vi "Execution Closed Event Callback.vi"(4 "TS UI Data":T1, 5 "Event Data":cluster{"exec":refnum<k7>}, 6 "Control Ref":refnum<k7>, 7 "Event Common Data":T2) -> ()   [LabVIEW 2015]
uses:
  Type defs/TS UI Data.ctl
  Type defs/Nest cluster.ctl
panel:
  # "SCANNED DATA"
  # "ITAC DATA"
  # "DoIP DATA"
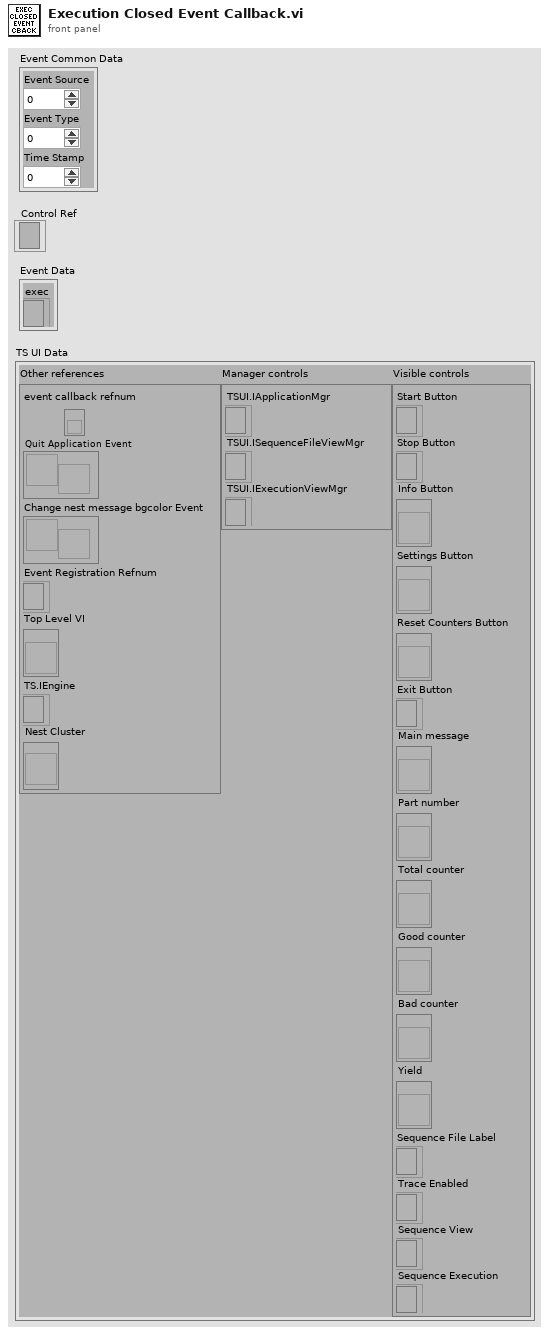
[diagram p1: front panel]
types:
  T1 = typedef "TS UI Data.ctl" = cluster{"Other references":cluster{"event callback refnum":refnum<k27>, "Quit Application Event":refnum<user-event>, "Change nest message bgcolor Event":refnum<user-event>, "event registration refnum":refnum<event-registration>, "Top Level VI":refnum<vi>, "TS.IEngine":refnum<k7>, "Nest Cluster":refnum<vi>}, "Manager controls":cluster{"TSUI.IApplicationMgr":refnum<k7>, "TSUI.ISequenceFileViewMgr":refnum<k7>, "TSUI.IExecutionViewMgr":refnum<k7>}, "Visible controls":cluster{"Start Button":refnum<k7>, "Stop Button":refnum<k7>, "Info Button":refnum<vi>, "Settings Button":refnum<vi>, "Reset Counters Button":refnum<vi>, "Exit Button":refnum<k7>, "Main message":refnum<vi>, "Part number":refnum<vi>, "Total counter":refnum<vi>, "Good counter":refnum<vi>, "Bad counter":refnum<vi>, "Yield":refnum<vi>, "Sequence File Label":refnum<k7>, "Trace Enabled":refnum<k7>, "Sequence View":refnum<k7>, "Sequence Execution":refnum<k7>}}
  T2 = cluster{"Event Source":i32, "Event Type":u32, "Time Stamp":u32}
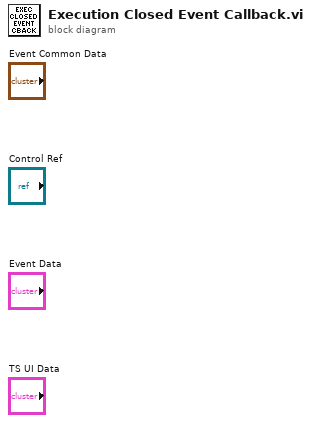
[diagram p0: block diagram]
diagram:
